vi "Before Iterative Write.vi"(8 "Error In":errorcluster, 10 "Temporary File":string, 11 "SFTP":refnum<class "SFTP.lvclass">) -> (0 "Error Out":errorcluster, 2 "Local":refnum<file>, 3 "SFTP File":refnum<class "SFTP File.lvclass">)   [LabVIEW 2018, in "Tests.lvlib" / "SFTP File.lvlib"]
uses:
  SFTP File.lvlib
  src/Toolkit/SFTP File/SFTP File.lvclass
  src/Toolkit/SFTP/SFTP.lvclass
  src/Toolkit/SFTP File/API/Typedefs/Flags.ctl
  src/Toolkit/Type Definitions/Permissions.ctl
  src/Toolkit/Type Definitions/Modes.ctl
  src/Toolkit/Toolkit.lvlib
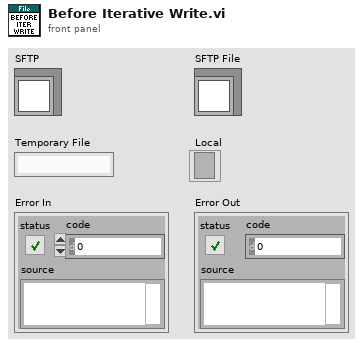
[diagram p1: front panel]
types:
  T1 = enum16{"open", "replace", "create", "open or create", "replace or create", "replace or create with confirmation"}
  T2 = typedef "Toolkit.lvlib/Permissions.ctl" = cluster{"Owner":T3, "Group":T3, "Others":T3}
  T3 = typedef "Toolkit.lvlib/Modes.ctl" = cluster{"Read":bool, "Write":bool, "Execute":bool}
  T4 = typedef "Toolkit.lvlib/SFTP File.lvclass/Flags.ctl" = cluster{"Read":bool, "Write":bool, "Append":bool, "Create":bool, "Truncate":bool, "Exclude":bool}
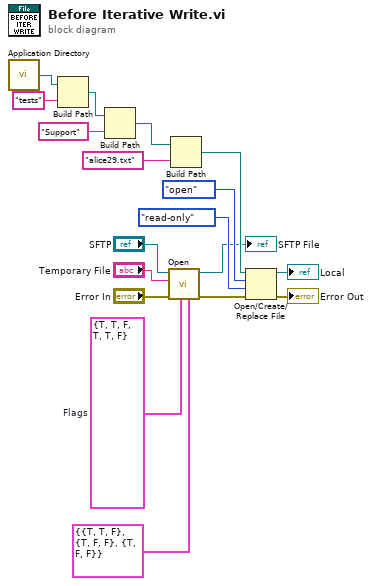
[diagram p0: block diagram]
diagram:
  w3 = T4 {"Read"=TRUE, "Write"=TRUE, "Append"=FALSE, "Create"=TRUE, "Truncate"=TRUE, "Exclude"=FALSE}  # Flags
  n1 = call <vilib>:"Application Directory.vi"() -> ("Application Directory"=w10:path)
  n2 = Build Path(base path=w10, name or relative path="tests") -> (appended path=w12:path)
  n3 = Build Path(base path=w12, name or relative path="Support") -> (appended path=w14:path)
  n4 = call "Open.vi"("Permissions"=T2 {"Owner"={"Read"=TRUE, "Write"=TRUE, "Execute"=FALSE}, "Group"={"Read"=TRUE, "Write"=FALSE, "Execute"=FALSE}, "Others"={"Read"=TRUE, "Write"=FALSE, "Execute"=FALSE}}, "Flags"=w3, "Error In"="Error In", "Remote Path"="Temporary File", "SFTP"="SFTP") -> ("Error Out"=w17:errorcluster, "SFTP File"=→"SFTP File":refnum<class "SFTP File.lvclass">)  [unwired: 5 in]
  n5 = Build Path(base path=w14, name or relative path="alice29.txt") -> (appended path=w15:path)
  n6 = Open/Create/Replace File(file path (use dialog)=w15, error in=w17, operation (0:open)=T1."open", access (0:read/write)=enum16{"read/write", "read-only", "write-only"}."read-only") -> (refnum out=→"Local":refnum<file>, error out=→"Error Out":errorcluster)  [unwired: 2 in, 1 out]
